vi "RSZVB Set UI Port Next State.vi"(8 "error in (no error)":errorcluster {"code" format="%.0x"}, 9 "Next State (0)":i32, 10 "Port (1)":i32=1, 11 "VISA session":refnum<visa-resource-name>) -> (0 "error out":errorcluster {"code" format="%.0x"}, 3 "dup VISA session":refnum<visa-resource-name>)   [LabVIEW 2011]
doc: "Defines the state of the output ports (pin 3 or 4) of the Universal Interface connector after the next negative pulse on the Input 1 line (pin 2). \n\nRemote-control command(s):\nCONTrol:HANDler:OUTPut<port>:USER"
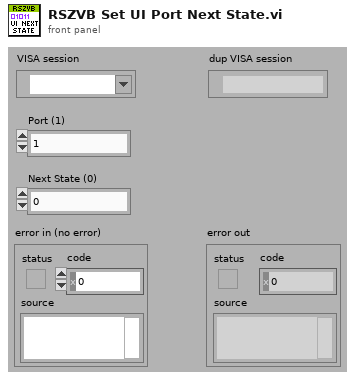
[diagram p1: front panel]
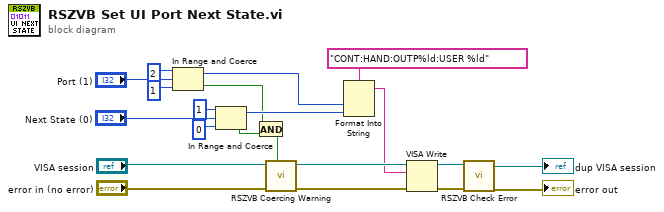
[diagram p0: block diagram]
diagram:
  n1 = In Range and Coerce(upper limit=2, x="Port (1)", lower limit=1) -> (coerced(x)=w7:i32, In Range?=w11:bool)
  n2 = In Range and Coerce(upper limit=1, x="Next State (0)", lower limit=0) -> (coerced(x)=w12:i32, In Range?=w10:bool)
  n3 = And(x=w11, y=w10) -> (x .and. y?=w9:bool)
  n4 = call "RSZVB Coercing Warning.vi"("In Range?"=w9, "error in (no error)"="error in (no error)", "VISA session"="VISA session") -> ("error out"=w18:errorcluster, "dup VISA session"=w19:refnum<visa-resource-name>)  [unwired: 7 in]
  n5 = Format Into String(format string="CONT:HAND:OUTP%ld:USER %ld", w7, w12) -> (resulting string=w15:string)  [unwired: 2 in, 1 out]
  n6 = VISA Write(VISA resource name=w19, write buffer=w15, error in (no error)=w18) -> (VISA resource name out=w16:refnum<visa-resource-name>, error out=w17:errorcluster)  [unwired: 1 out]
  n7 = call "RSZVB Check Error.vi"("error in (no error)"=w17, "VISA session"=w16) -> ("error out"=→"error out":errorcluster, "dup VISA session"=→"dup VISA session":refnum<visa-resource-name>)  [unwired: 8 in]
